vi "PRO_SwitchDetect.vi"(8 "SwP Threshold?":bool, 9 "Inputs":cluster{" Ohms":dbl, "Level OUt":dbl}, 10 "ChA Spec RNG In":T2, 11 "Switched In":bool) -> (2 "Level Out Def out":T1, 3 "Switched Out":bool)   [LabVIEW 2024]
uses:
  Control Definitions/Def_LevelSwitched.ctl
  Control Definitions/Def Spec RNG.ctl
  Control Definitions/Ded LUT_Status.ctl
panel:
  out "Boolean":bool
  in  "Level Out Def in":T1={"Switched"=FALSE, "Level OUt"=8.030499999999925, "Double Err"=FALSE}
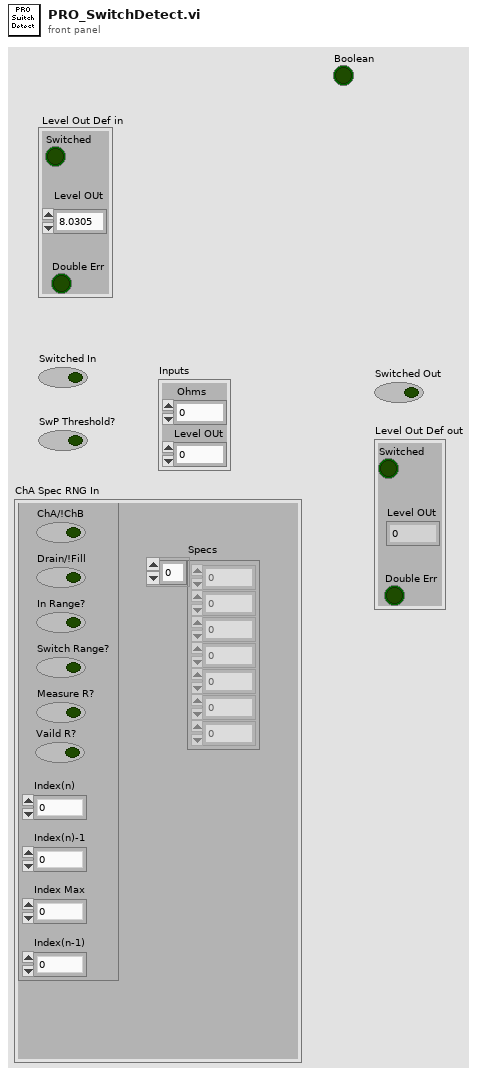
[diagram p1: front panel]
types:
  T1 = typedef "Def_LevelSwitched.ctl" = cluster{"Switched":bool, "Level OUt":dbl, "Double Err":bool}
  T2 = typedef "Def Spec RNG.ctl" = cluster{"Specs":dbl[], "LUT Status":T3}
  T3 = typedef "Ded LUT_Status.ctl" = cluster{"ChA/!ChB":bool, "Drain/!Fill":bool, "In Range?":bool, "Switch Range?":bool, "Measure R?":bool, "Vaild R?":bool, "Index(n)":i32, "Index(n)-1":i32, "Index Max":i32, "Index(n-1)":i32}
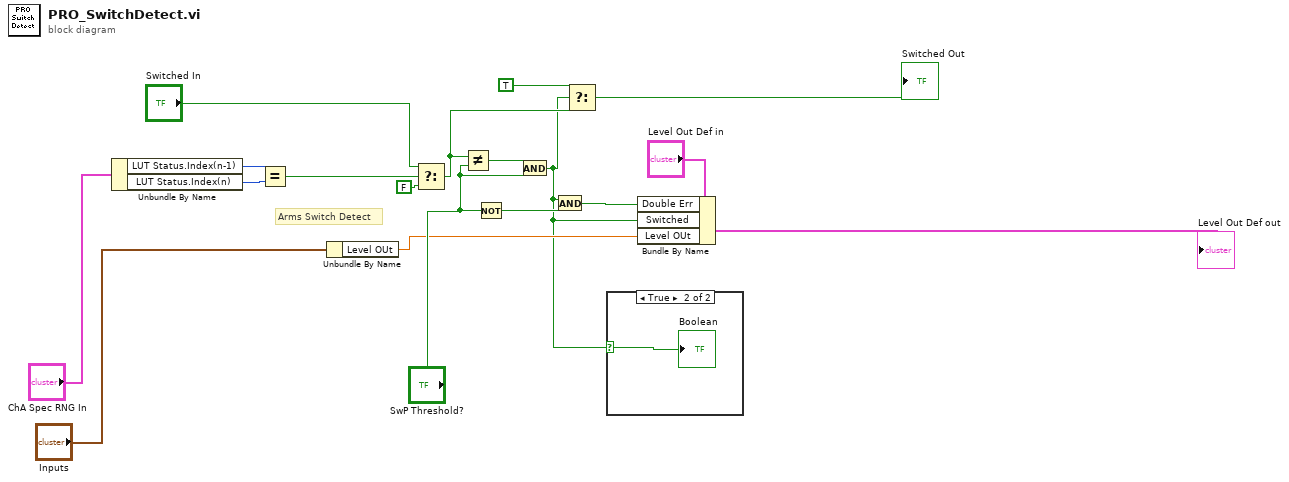
[diagram p0: block diagram]
diagram:
  # "Arms Switch Detect"
  n1 = Unbundle By Name("ChA Spec RNG In") -> ("LUT Status.Index(n-1)"=w8:i32, "LUT Status.Index(n)"=w9:i32)
  n2 = Equal?(x=w8, y=w9) -> (x = y?=w12:bool)
  n3 = Unbundle By Name("Inputs") -> ("Level OUt"=w11:dbl)
  n4 = Select(t="Switched In", s=w12, f=FALSE) -> (s? t:f=w15:bool)
  n5 = Not Equal?(x=w15, y="SwP Threshold?") -> (x != y?=w4:bool)
  n6 = Not(x="SwP Threshold?") -> (.not. x?=w17:bool)
  n7 = And(x=w4, y="SwP Threshold?") -> (x .and. y?=w1:bool)
  n8 = And(x=w1, y=w17) -> (x .and. y?=w2:bool)
  n9 = Select(t=TRUE, s=w1, f=w15) -> (s? t:f=→"Switched Out":bool)
  n10 = case shown="True" w1 {
    selector: w1 -> [_ w19]
    frame False {
    }
    frame True {
      "Boolean" <- w19
    }
  }
  n11 = Bundle By Name(cluster="Level Out Def in", "Double Err"=w2, "Switched"=w1, "Level OUt"=w11) -> (→"Level Out Def out":T1)
